vi "Connect COM Port & AutoBaud (SubVI).vi"(5 "Rx semaphore":T1, 7 "Tx semaphore":T1, 8 "error in (no error)":errorcluster, 10 "Rx":refnum<vi>, 11 "Tx":refnum<vi>) -> (0 "error out":errorcluster, 1 "BaudRate":string, 2 "Success?":bool caption="OK", 3 "VISA Refnum out":refnum<visa-resource-name>)   [LabVIEW 2017]
uses:
  <vilib>/Instr/_visa.llb/VISA Find Search Mode.ctl
  <vilib>/Instr/_visa.llb/VISA Configure Serial Port (Instr).vi
panel:
  in  "Baud rate":u32(ring)=8 items=["4800", "9600", "19200", "38400", "57600", "115200", "230400", "460800", "921600"]
  out "COM only list":string[](array[string])
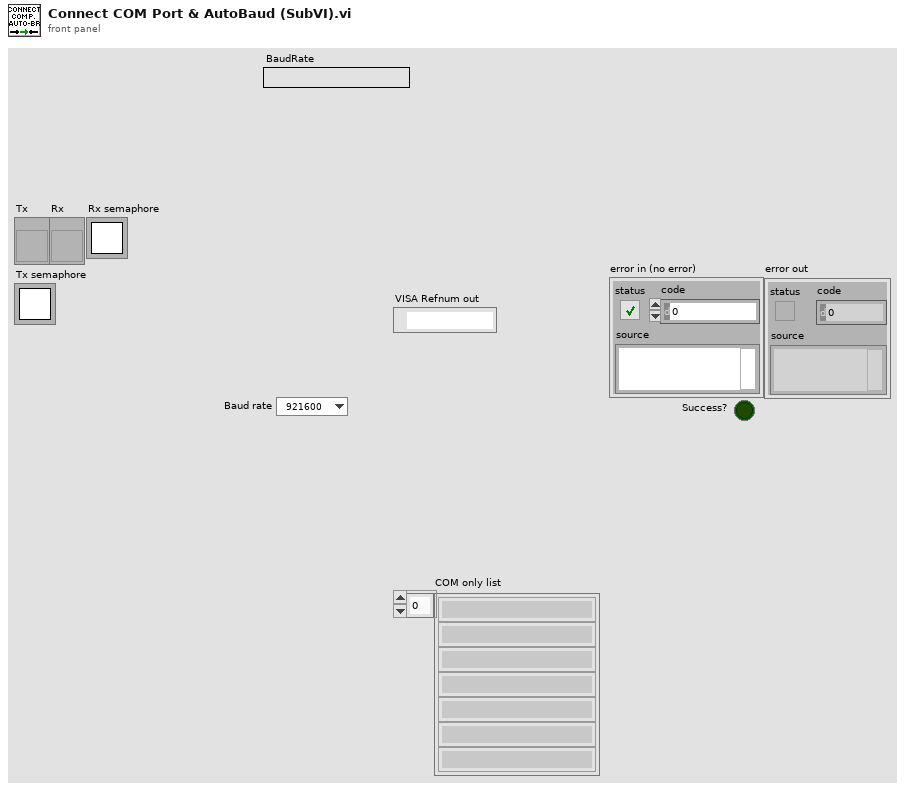
[diagram p1: front panel]
types:
  T1 = typedef "Semaphore RefNum" = refnum<k1>
  T2 = typedef "VISA Find Search Mode.ctl" = u32
  T3 = cluster{"Send Debug":string, "idx":u16, "DataType":enum8{"Int", " float"}, "Cmd id":u16, "Get/Set":enum8{"Set", "Get"}}
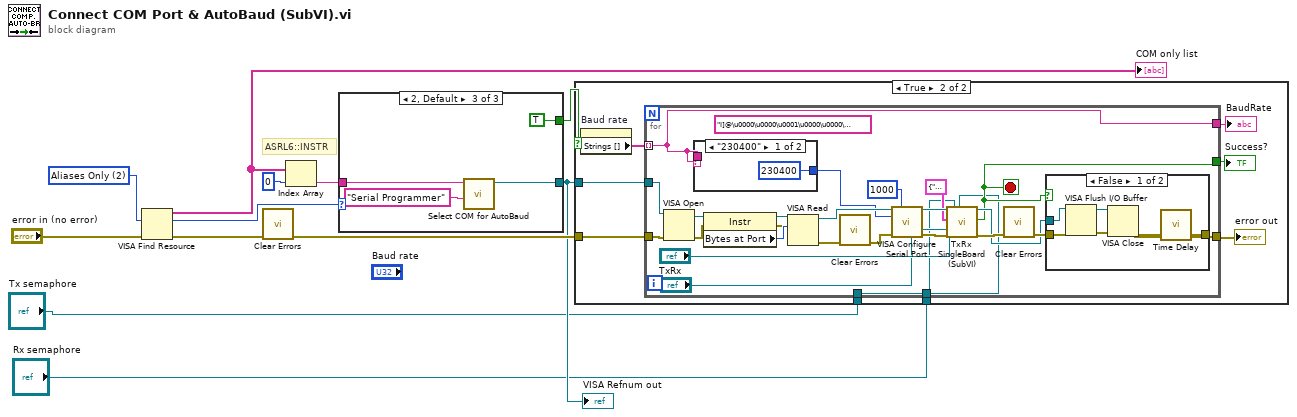
[diagram p0: block diagram]
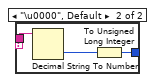
[diagram p3: hidden frame]
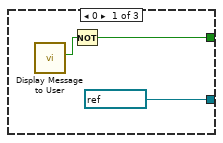
[diagram p5: hidden frame]
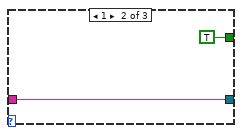
[diagram p6: hidden frame]
diagram:
  w6 = T2 2 items=["Canonical Names Only"=0, "Aliases Only"=2, "Include Matching Aliases"=3, "Include All Aliases"=4] ("Search Mode")
  # "ASRL6::INSTR"
  n1 = VISA Find Resource(8:"error in (no error)", 10:w6) -> (0:w11:errorcluster, 2:w7:u32, 3:w10:string[])  [unwired: 1 in]
  "COM only list" <- w10
  n2 = call <vilib>:"Clear Errors.vi"("error in (no error)"=w11) -> ("error out"=w8:errorcluster)  [unwired: 5 in, 1 out]
  n3 = Index Array(array=w10, index=0) -> (element=w5:string)
  n4 = case shown="2, Default" w7 {
    tunnel: [refnum<visa-resource-name> "COMx" ("VISA resource name out") w16 w20] -> w4
    tunnel: w5 -> [_ w16 w19]
    tunnel: [w15 TRUE TRUE] -> w3
    frame 0 {
      n5 = call "Display Message to User"() -> ("OK"=w13:bool)  [unwired: 10 in, 1 out]
      n6 = Not(x=w13) -> (.not. x?=w15:bool)
    }
    frame 1 {
    }
    frame 2, Default {
      n7 = call "Select COM for AutoBaud.vi"("Port Name"="Serial Programmer", "VISA resource name 2"=w19) -> ("VISA resource name out"=w20:refnum<visa-resource-name>)  [unwired: 7 in, 2 out]
    }
  }
  "VISA Refnum out" <- w4
  n8 = case shown="True" w3 {
    tunnel: w4 -> [_ w29]
    tunnel: w8 -> [_ w28]
    tunnel: "Tx semaphore" -> [_ w24]
    tunnel: "Rx semaphore" -> [_ w23]
    frame False {
    }
    frame True {
      n9 = property on="Baud rate" class="Ring (strict)"() -> ("Strings []"=w27:string[])  [unwired: 2 in, 2 out]
      n10 = for {
        tunnel: w29 -> [w52]
        tunnel: w28 -> [w51]
        tunnel: [w47] -> w26
        tunnel: w27 -> [w31] mode=indexing
        tunnel: [w46] -> w25
        tunnel: w24 -> [w42]
        tunnel: w23 -> [w41]
        tunnel: [w31] -> w22
        stop <- w46 stop-if-true
        (unwired) "I]@\u0000\u0000\u0001\u0000\u0000\u0000@8" ("MessageToSend")
        n11 = VISA Open(error in (no error)=w51, VISA resource name=w52) -> (VISA resource name=w39:refnum<visa-resource-name>, error out=w38:errorcluster)  [unwired: 3 in]
        n12 = case shown="\"230400\"" w31 {
          tunnel: w31 -> [_ w57]
          tunnel: [u32 230400 w56] -> w32
          frame "230400" {
          }
          frame "\u0000", Default {
            n13 = Decimal String To Number(string=w57) -> (number=w58:i32)  [unwired: 2 in, 1 out]
            n14 = To Unsigned Long Integer(number=w58) -> (unsigned 32bit integer=w56:u32)
          }
        }
        n15 = property class="Instr"(reference=w39, error in=w38) -> (reference out=w36:refnum<visa-resource-name>, error out=w35:errorcluster, "Bytes at Port"=w37:u32)
        n16 = VISA Read(VISA resource name=w36, byte count=w37, error in (no error)=w35) -> (VISA resource name out=w33:refnum<visa-resource-name>, error out=w34:errorcluster)  [unwired: 2 out]
        n17 = call <vilib>:"Clear Errors.vi"("error in (no error)"=w34) -> ("error out"=w30:errorcluster)  [unwired: 5 in, 1 out]
        n18 = call-poly "VISA Configure Serial Port"("VISA resource name"=w33, "timeout (10sec)"=u32 1000, "baud rate (9600)"=w32, "error in (no error)"=w30) -> ("VISA resource name out"=w54:refnum<visa-resource-name>, "error out"=w53:errorcluster)  [unwired: 10 in]
        n19 = call "TxRx SingleBoard (SubVI).vi"("VISA Refnum in"=w54, "DataMessage Tx"=T3 {"Send Debug"="1", "idx"=0, "DataType"=enum."Int", "Cmd id"=64, "Get/Set"=enum."Set"} ("DataMessage"), "Tx"="Tx", "Rx"="Rx", "error in (no error)"=w53, "Tx semaphore"=w42, "Rx semaphore"=w41) -> ("VISA Refnum out"=w48:refnum<visa-resource-name>, "DataReceived?"=w46:bool, "error out"=w50:errorcluster)  [unwired: 6 in, 4 out]
        n20 = call <vilib>:"Clear Errors.vi"("error in (no error)"=w50) -> ("error out"=w49:errorcluster)  [unwired: 5 in, 1 out]
        n21 = case shown="False" w46 {
          tunnel: w49 -> [w64 w65]
          tunnel: w48 -> [w61 _]
          tunnel: [w60 w65] -> w47
          frame False {
            n22 = VISA Flush I/O Buffer(VISA resource name=w61, error in (no error)=w64) -> (VISA resource name out=w62:refnum<visa-resource-name>, error out=w63:errorcluster)  [unwired: 1 in]
            n23 = VISA Close(VISA resource name=w62, error in (no error)=w63) -> (error out=w59:errorcluster)
            n24 = call "Time Delay"("error in (no error)"=w59) -> ("error out"=w60:errorcluster)  [unwired: 10 in]
          }
          frame True {
          }
        }
      }
      "error out" <- w26
      "Success?" <- w25
      "BaudRate" <- w22
    }
  }
